vi "De-Block and Reverse Data Set.vi"(9 "Pos to Start Scan":i32=10000, 10 "data value reference":refnum<data-value>, 11 "Final No of Blocks":i32) -> (2 "data value ref out":refnum<data-value>)   [LabVIEW 2015, in "Tool Module.lvlib"]
uses:
  Tool Module.lvlib
  ToolModGLOB.vi
  Tool Config/Tool Cfg.lvlib
panel:
  in  "error in (no error)":errorcluster
  out "error out":errorcluster
  out "Sample Count Graph":u32[](graph)
  out "Axial Pos Array":dbl[](array[numeric])
  out "Reversed Array out":u32[][](array[numeric])
  in  "Scan Data Array in":u32[][](array[numeric])=[[0, 1, 2, 3, 4, 5], [10, 11, 12, 13, 14, 15], [20, 21, 22, 23, 24, 25], [30, 31, 32, 33, 34, 35], [40, 41, 42, 43, 44, 45]]
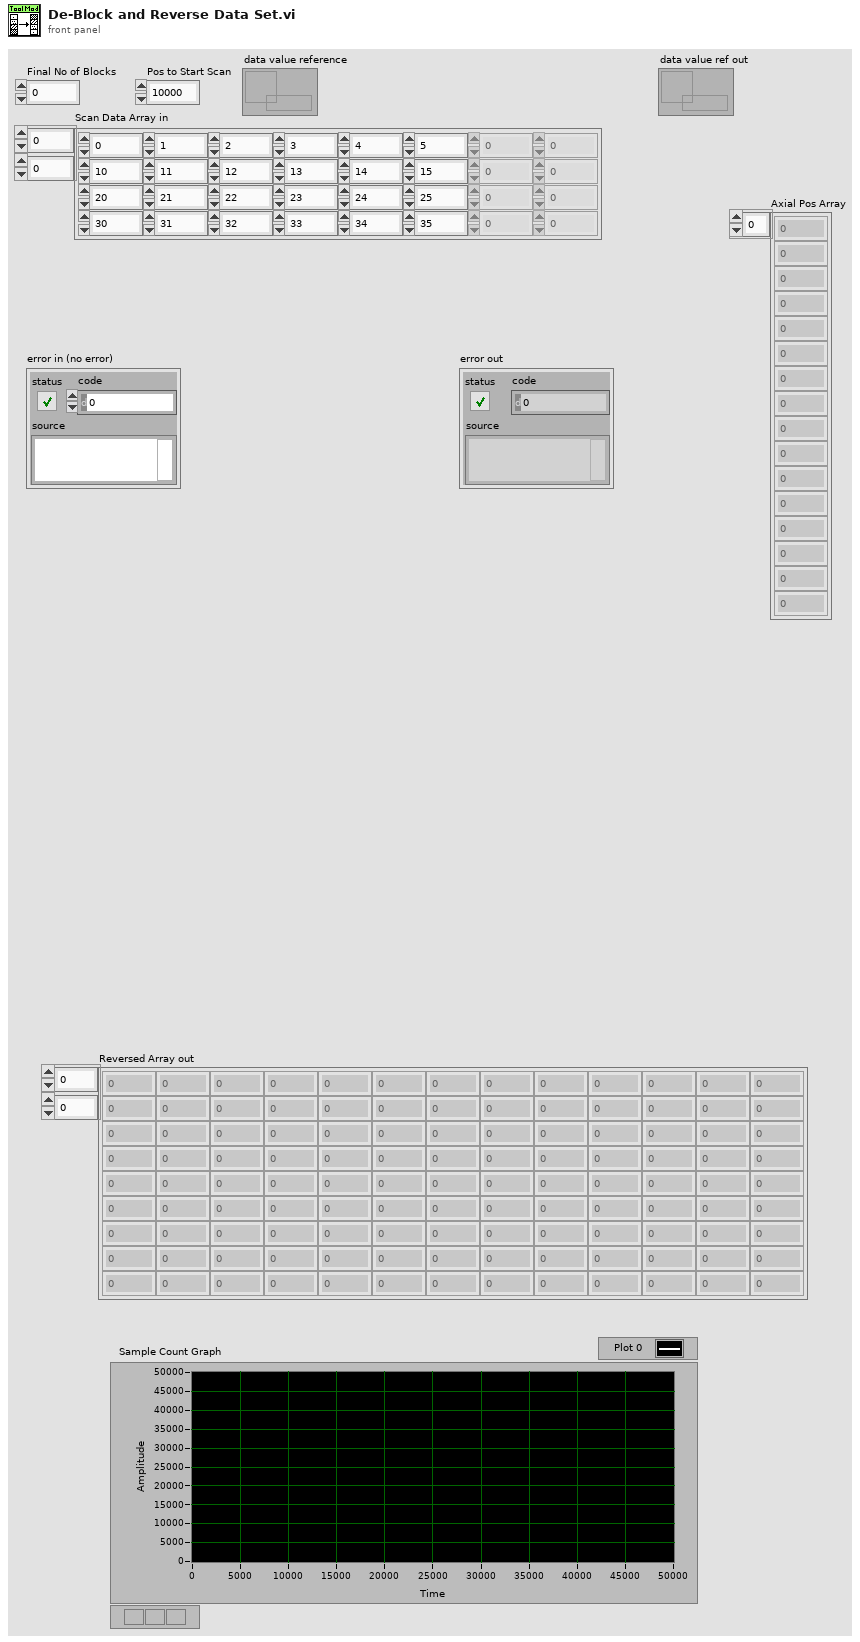
[diagram p1: front panel]
types:
  T1 = typedef "_Data Stream Fmt Params Cluster--typedef.ctl" = cluster{"Samples per Block":i32, "Raw Data Status Len":i32, "Fltr Data Status Len":i32}
  T2 = typedef "Tool Cfg.lvlib/_Tool Operation Config Cluster--typedef.ctl" = cluster{"Use Tool Cfg":bool, "Use Tool Cal":bool, "Fake Data?":bool, "Mode":i16, "Array Subset Length":i16, "nArrays to Read":i16, "Full Array Read Length":i16, "nSubarrays/Sensor":i16}
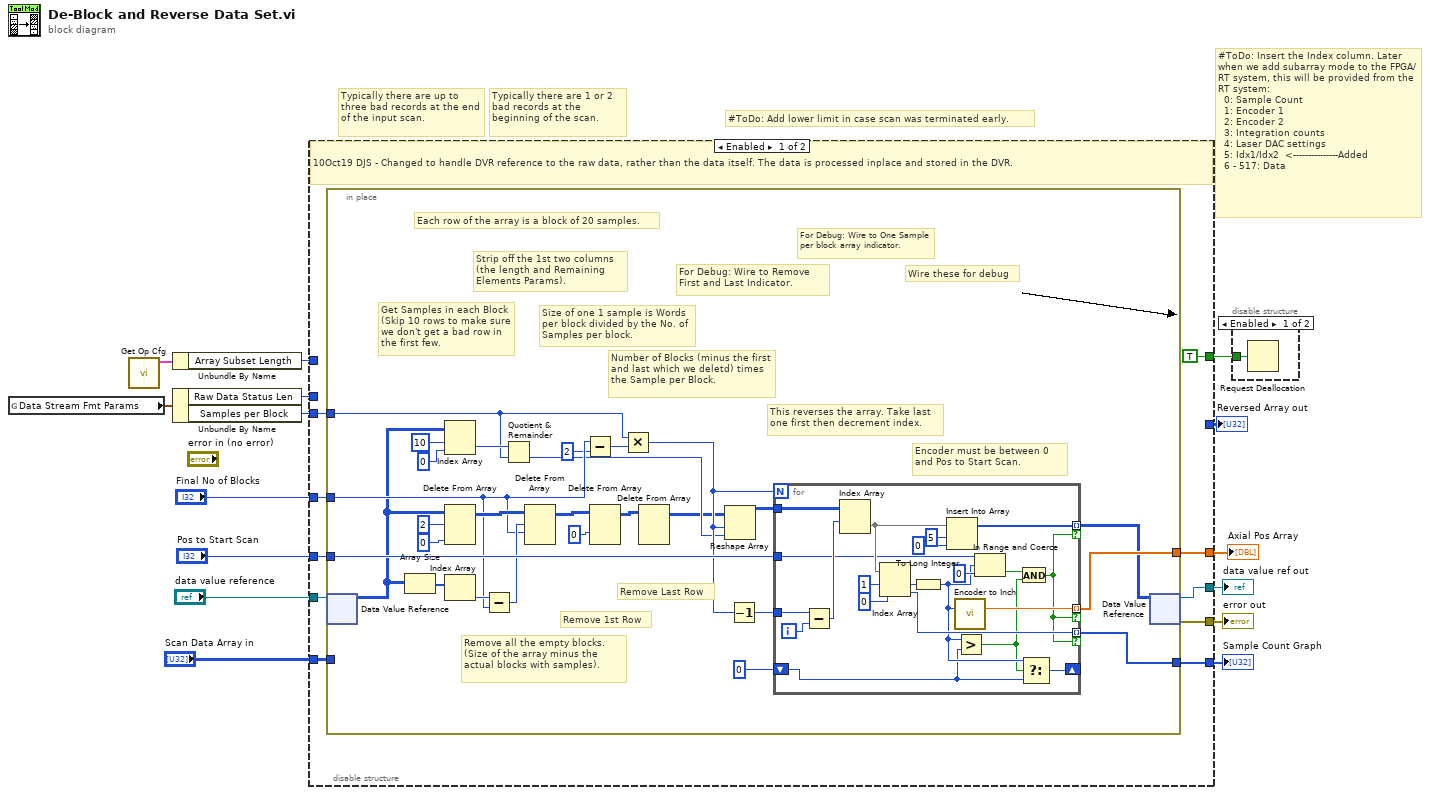
[diagram p0: block diagram]
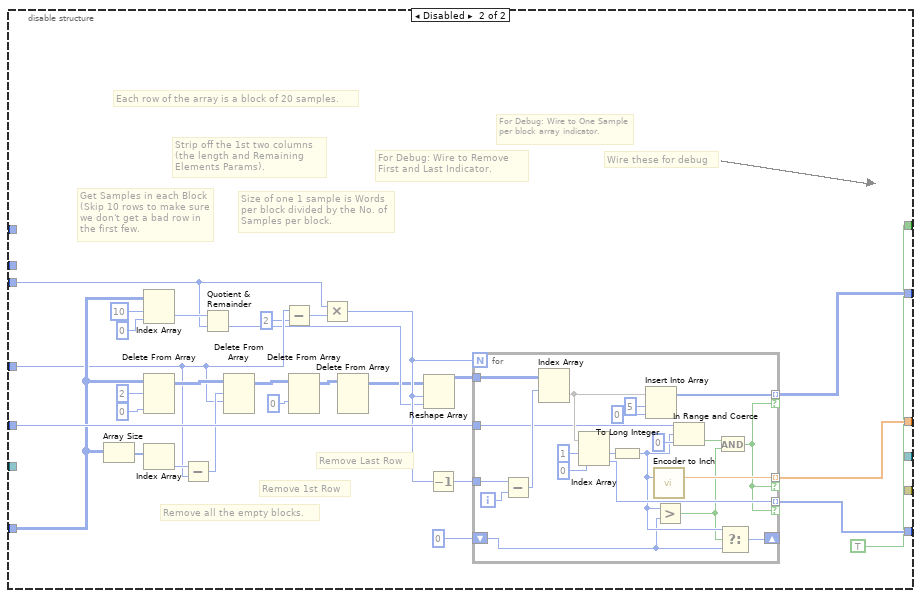
[diagram p2: hidden frame]
diagram:
  # "#ToDo: Insert the Index column. Later when we add subarray mode to the FPGA/RT system, this will be provided from the RT system:\n  0: Sample Count\n  1: Encoder 1\n  2: Encoder 2\n  3: Integration counts\n  4: Laser DAC settings\n  5: Idx1/Idx2  <---------------Added\n  6 - 517: Data"
  # "#ToDo: Add lower limit in case scan was terminated early."
  # "Typically there are 1 or 2 bad records at the beginning of the scan."
  # "Typically there are up to three bad records at the end of the input scan."
  n1 = global read "ToolModGLOB.vi" "Data Stream Fmt Params"() -> (w14:T1)
  n2 = call "Get Op Cfg.vi"() -> ("Tool Operation Config"=w12:T2)  [unwired: 11 in]
  n3 = Unbundle By Name(w12) -> ("Array Subset Length"=w11:i16)
  n4 = Unbundle By Name(w14) -> ("Raw Data Status Len"=w13:i32, "Samples per Block"=w10:i32)
  n5 = disable-structure shown="Enabled" {
    disable-tunnel: "Final No of Blocks" -> [w23 w87]
    disable-tunnel: "Scan Data Array in" -> [w24 w93]
    disable-tunnel: w13 -> [_ _]
    disable-tunnel: w11 -> [_ _]
    disable-tunnel: w10 -> [w22 w85]
    disable-tunnel: "Pos to Start Scan" -> [w25 w95]
    disable-tunnel: [_ w83] -> w8
    disable-tunnel: [w20 w75] -> w6
    disable-tunnel: [w21 w76] -> w5
    disable-tunnel: [TRUE TRUE] -> w4
    disable-tunnel: "data value reference" -> [w17 _]
    disable-tunnel: [w18 _] -> w2
    disable-tunnel: [w16 _] -> w1
    frame Enabled {
      # "10Oct19 DJS - Changed to handle DVR reference to the raw data, rather than the data itself. The data is processed inplace and stored in the DVR."
      n6 = in-place {
        in-place-border: w25 -> [w46]
        in-place-border: w24 -> [_]
        in-place-border: w23 -> [w39]
        in-place-border: w22 -> [w37]
        in-place-border: [w29] -> w21
        in-place-border: [w28] -> w20
        # "Number of Blocks (minus the first and last which we deletd) times the Sample per Block."
        # "Encoder must be between 0 and Pos to Start Scan."
        # "This reverses the array. Take last one first then decrement index."
        # "Each row of the array is a block of 20 samples."
        # "Size of one 1 sample is Words per block divided by the No. of Samples per block."
        # "Get Samples in each Block (Skip 10 rows to make sure we don't get a bad row in the first few."
        # "Remove all the empty blocks. (Size of the array minus the actual blocks with samples)."
        # "Strip off the 1st two columns (the length and Remaining Elements Params)."
        # "For Debug: Wire to One Sample per block array indicator."
        # "For Debug: Wire to Remove First and Last Indicator."
        # "Wire these for debug"
        # "Remove Last Row"
        # "Remove 1st Row"
        n7 = in-place-dvr #1(w17) -> (w27:u32[][])  [unwired: 1 out]
        n8 = Array Size(array=w27) -> (size(s)=w44:i32[])
        n9 = Index Array(array=w27, index (row)=10, index (col)=0 ("disabled index (col)")) -> (element=w52:u32)
        n10 = Delete From Array(array=w27, length=2, index (col)=0 ("disabled index (col)")) -> (array with subset deleted=w45:u32[][])  [unwired: 1 in, 1 out]
        n11 = Index Array(array=w44) -> (element=w43:i32)  [unwired: 1 in]
        n12 = Subtract(x=w43, y=w39) -> (x-y=w42:i32)
        n13 = Quotient & Remainder(x=w52, y=w37) -> (floor(x/y)=w32:u32)  [unwired: 1 out]
        n14 = Delete From Array(array=w45, length=w42, index (row)=w39) -> (array with subset deleted=w36:u32[][])  [unwired: 1 in, 1 out]
        n15 = Subtract(x=w39, y=2) -> (x-y=w34:i32)
        n16 = Delete From Array(array=w36, index (row)=0) -> (array with subset deleted=w40:u32[][])  [unwired: 2 in, 1 out]
        n17 = Multiply(x=w37, y=w34) -> (x*y=w33:i32)
        n18 = Delete From Array(array=w40) -> (array with subset deleted=w30:u32[][])  [unwired: 3 in, 1 out]
        n19 = Reshape Array(w30, w33, w32) -> (w35:u32[][])
        n20 = Decrement(x=w33) -> (x-1=w47:i32)
        n21 = for {
          N: w33 -> [_]
          tunnel: w35 -> [w73]
          tunnel: w47 -> [w70]
          tunnel: [w63] -> w26 mode=indexing if=w54
          tunnel: w46 -> [w65]
          tunnel: [w66] -> w29 mode=indexing if=w54
          tunnel: [w59] -> w28 mode=indexing if=w54
          shift-right: [w57] -> _
          shift-left: 0 -> [w55]
          i -> [w71]
          n22 = Subtract(x=w70, y=w71) -> (x-y=w72:i32)
          n23 = Index Array(array=w73, index (row)=w72) -> (element=w69:u32[])  [unwired: 1 in]
          n24 = Index Array(array=w69, index #1=1 ("index"), index #2=0 ("index")) -> (element #1=w68:u32, element #2=w59:u32)
          n25 = To Long Integer(number=w68) -> (32bit integer=w56:i32)
          n26 = Insert Into Array(array=w69, index=5, new element=u32 0 ("new element/subarray")) -> (w63:u32[])
          n27 = call "Encoder to Inch.vi"("Encoder in"=w56) -> ("Encoder out(in)"=w66:dbl)  [unwired: 14 in]
          n28 = Greater?(x=w56, y=w55) -> (0:w53:bool)
          n29 = In Range and Coerce(upper limit=w65, x=w56, lower limit=0) -> (In Range?=w58:bool)  [unwired: 1 out]
          n30 = And(x=w58, y=w53) -> (x .and. y?=w54:bool)
          n31 = Select(t=w56, s=w53, f=w55) -> (s? t:f=w57:i32)
        }
        n32 = in-place-dvr #1(w26) -> (w18:refnum<data-value>, w16:errorcluster)
      }
    }
    frame Disabled {
      # "Each row of the array is a block of 20 samples."
      # "Size of one 1 sample is Words per block divided by the No. of Samples per block."
      # "Get Samples in each Block (Skip 10 rows to make sure we don't get a bad row in the first few."
      # "Remove all the empty blocks."
      # "Strip off the 1st two columns (the length and Remaining Elements Params)."
      # "For Debug: Wire to One Sample per block array indicator."
      # "For Debug: Wire to Remove First and Last Indicator."
      # "Wire these for debug"
      # "Remove Last Row"
      # "Remove 1st Row"
      n33 = Array Size(array=w93) -> (size(s)=w92:i32[])
      n34 = Index Array(array=w93, index (row)=10, index (col)=0 ("disabled index (col)")) -> (element=w101:u32)
      n35 = Delete From Array(array=w93, length=2, index (col)=0 ("disabled index (col)")) -> (array with subset deleted=w94:u32[][])  [unwired: 1 in, 1 out]
      n36 = Index Array(array=w92) -> (element=w91:i32)  [unwired: 1 in]
      n37 = Subtract(x=w91, y=w87) -> (x-y=w90:i32)
      n38 = Quotient & Remainder(x=w101, y=w85) -> (floor(x/y)=w79:u32)  [unwired: 1 out]
      n39 = Delete From Array(array=w94, length=w90, index (row)=w87) -> (array with subset deleted=w84:u32[][])  [unwired: 1 in, 1 out]
      n40 = Subtract(x=w87, y=2) -> (x-y=w81:i32)
      n41 = Delete From Array(array=w84, index (row)=0) -> (array with subset deleted=w88:u32[][])  [unwired: 2 in, 1 out]
      n42 = Multiply(x=w85, y=w81) -> (x*y=w80:i32)
      n43 = Delete From Array(array=w88) -> (array with subset deleted=w77:u32[][])  [unwired: 3 in, 1 out]
      n44 = Reshape Array(w77, w80, w79) -> (w82:u32[][])
      n45 = Decrement(x=w80) -> (x-1=w96:i32)
      n46 = for {
        N: w80 -> [_]
        tunnel: w82 -> [w122]
        tunnel: w96 -> [w119]
        tunnel: [w112] -> w83 mode=indexing if=w103
        tunnel: w95 -> [w114]
        tunnel: [w115] -> w76 mode=indexing if=w103
        tunnel: [w108] -> w75 mode=indexing if=w103
        shift-right: [w106] -> _
        shift-left: 0 -> [w104]
        i -> [w120]
        n47 = Subtract(x=w119, y=w120) -> (x-y=w121:i32)
        n48 = Index Array(array=w122, index (row)=w121) -> (element=w118:u32[])  [unwired: 1 in]
        n49 = Index Array(array=w118, index #1=1 ("index"), index #2=0 ("index")) -> (element #1=w117:u32, element #2=w108:u32)
        n50 = To Long Integer(number=w117) -> (32bit integer=w105:i32)
        n51 = Insert Into Array(array=w118, index=5, new element=u32 0 ("new element/subarray")) -> (w112:u32[])
        n52 = call "Encoder to Inch.vi"("Encoder in"=w105) -> ("Encoder out(in)"=w115:dbl)  [unwired: 14 in]
        n53 = Greater?(x=w105, y=w104) -> (0:w102:bool)
        n54 = In Range and Coerce(upper limit=w114, x=w105, lower limit=0) -> (In Range?=w107:bool)  [unwired: 1 out]
        n55 = And(x=w107, y=w102) -> (x .and. y?=w103:bool)
        n56 = Select(t=w105, s=w102, f=w104) -> (s? t:f=w106:i32)
      }
    }
  }
  "Reversed Array out" <- w8
  "Axial Pos Array" <- w5
  "Sample Count Graph" <- w6
  "data value ref out" <- w2
  "error out" <- w1
  n57 = disable-structure shown="Enabled" {
    disable-tunnel: w4 -> [w123 _]
    frame Enabled {
      n58 = Request Deallocation(w123) -> ()
    }
    frame Disabled {
    }
  }
